vi "Scale.vi"(7 "Relative?":bool, 8 "error in (no error)":errorcluster, 10 "Scale":cluster{"X":sgl, "Y":sgl, "Z":sgl}, 11 "3D Object in":refnum<class "3D Object.lvclass">) -> (0 "error out":errorcluster, 3 "3D Object out":refnum<class "3D Object.lvclass">)   [LabVIEW 2015, in "3D Object.lvclass"]
uses:
  3D Object.lvclass
  3D Object.lvclass/3D Object.ctl
  <vilib>/picture/3D Picture Control/NI_3D Picture Control.lvlib
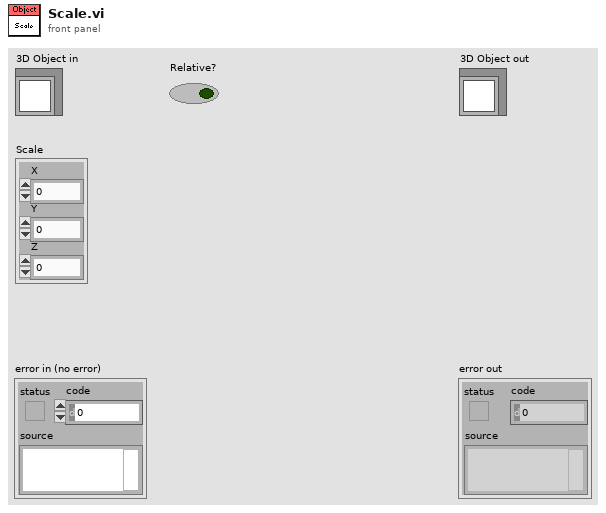
[diagram p1: front panel]
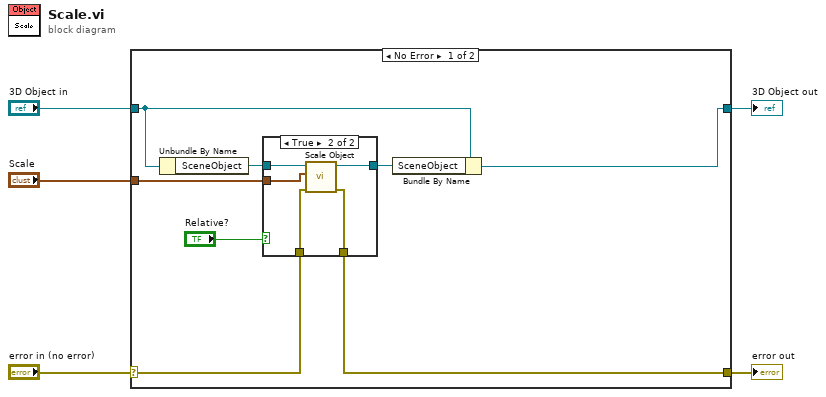
[diagram p0: block diagram]
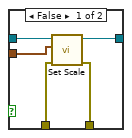
[diagram p2: hidden frame]
diagram:
  n1 = case shown="No Error" "error in (no error)" {
    selector: "error in (no error)" -> [w12 w25]
    tunnel: [w11 w25] -> w4
    tunnel: [w8 w24] -> w2
    tunnel: "3D Object in" -> [w9 w24]
    tunnel: "Scale" -> [w10 _]
    frame No Error {
      n2 = Unbundle By Name(w9) -> ("SceneObject"=w13:refnum<vi>)
      n3 = case shown="True" "Relative?" {
        tunnel: w13 -> [w18 w23]
        tunnel: w12 -> [w17 w22]
        tunnel: [w16 w21] -> w11
        tunnel: w10 -> [w15 w20]
        tunnel: [w14 w19] -> w7
        frame False {
          n4 = call <vilib>:"Set Scale.vi"("error in (no error)"=w17, "Scale"=w15, "Scene Object"=w18) -> ("error out"=w16:errorcluster, "Scaled Object"=w14:refnum<vi>)  [unwired: 7 in]
        }
        frame True {
          n5 = call <vilib>:"Scale Object.vi"("error in (no error)"=w22, "Scale"=w20, "Scene.Object In"=w23) -> ("error out"=w21:errorcluster, "Scene.Object Out"=w19:refnum<vi>)  [unwired: 7 in]
        }
      }
      n6 = Bundle By Name(cluster=w9, "SceneObject"=w7) -> (w8:refnum<class "3D Object.lvclass">)
    }
    frame Error {
    }
  }
  "error out" <- w4
  "3D Object out" <- w2
